vi "VISA_ListDevice.vi"(8 "error in (no error)":errorcluster) -> (0 "error out":errorcluster, 3 "find list":string[](array[string])=["ASRL1::INSTR", "ASRL2::INSTR", "ASRL3::INSTR"])   [LabVIEW 2014, in "QwaveSys Raspberry Pi Library.lvlib"]
uses:
  <vilib>/Instr/_visa.llb/VISA Find Search Mode.ctl
  QwaveSys Raspberry Pi Library.lvlib
panel:
  out "return count":u32=3
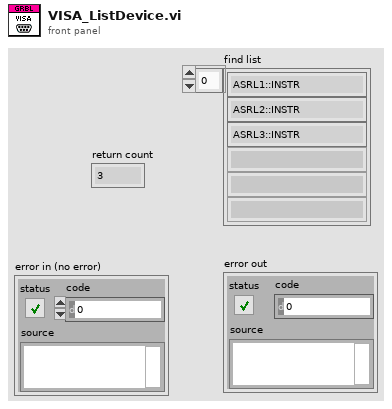
[diagram p1: front panel]
types:
  T1 = typedef "VISA Find Search Mode.ctl" = u32
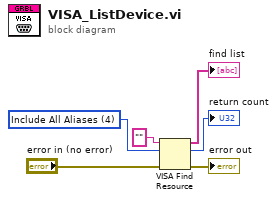
[diagram p0: block diagram]
diagram:
  w5 = T1 4 items=["Canonical Names Only"=0, "Aliases Only"=2, "Include Matching Aliases"=3, "Include All Aliases"=4] ("Search Mode")
  n1 = VISA Find Resource(8:"error in (no error)", 10:w5, 11:"" ("expression (\"?*\")")) -> (0:→"error out":errorcluster, 2:→"return count":u32, 3:→"find list":string[])
